vi "Direction To Angle.vi"(11 "Direction":T1) -> (3 "angle (deg)":dbl)   [LabVIEW 2020, in "DS Square.lvlib"]
uses:
  DS Square.lvlib
  Type Defs/Direction Enum.ctl
  Type Defs/SB Type Defs.lvlib
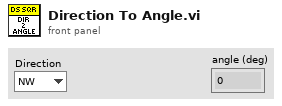
[diagram p1: front panel]
types:
  T1 = typedef "SB Type Defs.lvlib/Direction Enum.ctl" = enum16{"NW", "N", "NE", "E", "SE", "S", "SW", "W"}
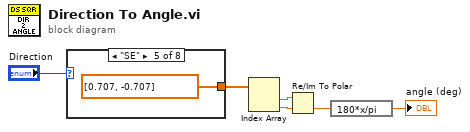
[diagram p0: block diagram]
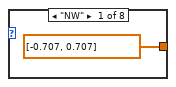
[diagram p2: hidden frame]
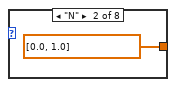
[diagram p3: hidden frame]
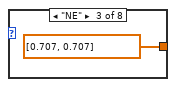
[diagram p4: hidden frame]
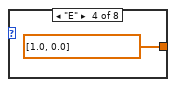
[diagram p5: hidden frame]
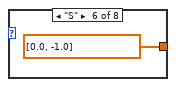
[diagram p6: hidden frame]
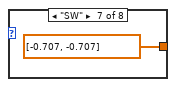
[diagram p7: hidden frame]
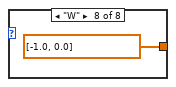
[diagram p8: hidden frame]
diagram:
  n1 = case shown="\"SE\"" "Direction" {
    tunnel: [dbl[] [-0.707, 0.707] ("X Vector") dbl[] [0.0, 1.0] ("X Vector") dbl[] [0.707, 0.707] ("X Vector") dbl[] [1.0, 0.0] ("X Vector") dbl[] [0.707, -0.707] ("X Vector") dbl[] [0.0, -1.0] ("X Vector") dbl[] [-0.707, -0.707] ("X Vector") dbl[] [-1.0, 0.0] ("X Vector")] -> w5
    frame "NW" {
    }
    frame "N" {
    }
    frame "NE" {
    }
    frame "E" {
    }
    frame "SE" {
    }
    frame "S" {
    }
    frame "SW" {
    }
    frame "W" {
    }
  }
  n2 = Index Array(array=w5) -> (element #1=w4:dbl, element #2=w3:dbl)  [unwired: 2 in]
  n3 = Re/Im To Polar(2:w3, 3:w4) -> (0:w2:dbl)  [unwired: 1 out]
  n4 = expression code="180*x/pi"(w2) -> (→"angle (deg)":dbl)
